vi "Design Lowpass Filter.vi"(10 "Conversion Op":T1, 11 "dt":dbl) -> (3 "filter coefficients":cluster{"beta":dbl, "gamma":dbl, "alpha":dbl} {"alpha" format="%.2f"; "gamma" format="%.2f"; "beta" format="%.2f"})   [LabVIEW 2017, in "VibrationAnalysisFunctions.lvlib"]
uses:
  <vilib>/addons/InsightCM/Utilities/Analysis/Vibration/VibrationAnalysisFunctions.lvlib
  <vilib>/addons/InsightCM/Utilities/Analysis/Shared/controls/ConversionOp.ctl
  <vilib>/addons/InsightCM/Utilities/Analysis/Shared/AnalysisHelper.lvlib
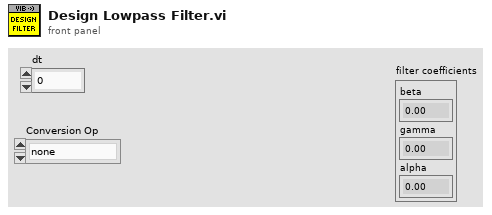
[diagram p1: front panel]
types:
  T1 = typedef "AnalysisHelper.lvlib/ConversionOp.ctl" = enum16{"none", "singleInt", "doubleInt", "singleDiff", "doubleDiff"}
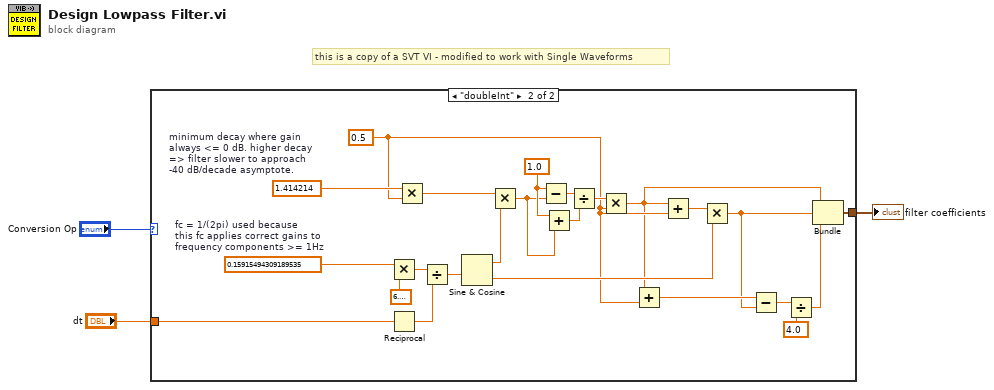
[diagram p0: block diagram]
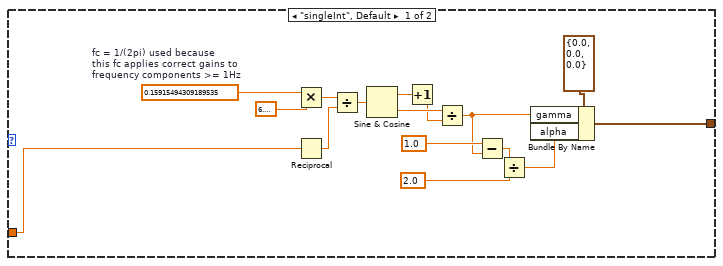
[diagram p2: hidden frame]
diagram:
  # "this is a copy of a SVT VI - modified to work with Single Waveforms"
  n1 = case shown="\"doubleInt\"" "Conversion Op" {
    tunnel: [w4 w21] -> w3
    tunnel: "dt" -> [w5 w20]
    frame "singleInt", Default {
      w19 = 0.15915494309189535  # fc = 1/(2pi) used because  this fc applies correct gains to  frequency components >= 1Hz
      n2 = Multiply(x=w19, y=6.283185307179586) -> (x*y=w13:dbl)
      n3 = Reciprocal(x=w5) -> (1/x=w14:dbl)
      n4 = Divide(x=w13, y=w14) -> (x/y=w12:dbl)
      n5 = Sine & Cosine(0:w12) -> (1:w17:dbl, 2:w16:dbl)
      n6 = Increment(x=w17) -> (x+1=w15:dbl)
      n7 = Divide(x=w16, y=w15) -> (x/y=w7:dbl)
      n8 = Subtract(x=1.0, y=w7) -> (x-y=w10:dbl)
      n9 = Divide(x=w10, y=2.0) -> (x/y=w6:dbl)
      n10 = Bundle By Name(cluster=cluster{"beta":dbl, "gamma":dbl, "alpha":dbl} {"beta"=0.0, "gamma"=0.0, "alpha"=0.0} ("filter coefficients"), "gamma"=w7, "alpha"=w6) -> (w4:cluster{"beta":dbl, "gamma":dbl, "alpha":dbl})
    }
    frame "doubleInt" {
      w25 = 0.5 ("y")
      w35 = 1.0 ("x")
      w41 = 1.414214  # minimum decay where gain  always <= 0 dB. higher decay => filter slower to approach  -40 dB/decade asymptote.
      w42 = 0.15915494309189535  # fc = 1/(2pi) used because  this fc applies correct gains to  frequency components >= 1Hz
      n11 = Multiply(x=w42, y=6.283185307179586) -> (x*y=w39:dbl)
      n12 = Reciprocal(x=w20) -> (1/x=w24:dbl)
      n13 = Multiply(x=w41, y=w25) -> (x*y=w37:dbl)
      n14 = Divide(x=w39, y=w24) -> (x/y=w38:dbl)
      n15 = Sine & Cosine(0:w38) -> (1:w36:dbl, 2:w29:dbl)
      n16 = Multiply(x=w37, y=w36) -> (x*y=w34:dbl)
      n17 = Subtract(x=w35, y=w34) -> (x-y=w33:dbl)
      n18 = Add(x=w35, y=w34) -> (x+y=w32:dbl)
      n19 = Divide(x=w33, y=w32) -> (x/y=w31:dbl)
      n20 = Multiply(x=w31, y=w25) -> (x*y=w22:dbl)
      n21 = Add(x=w22, y=w25) -> (x+y=w28:dbl)
      n22 = Add(x=w22, y=w25) -> (x+y=w30:dbl)
      n23 = Multiply(x=w30, y=w29) -> (x*y=w23:dbl)
      n24 = Subtract(x=w28, y=w23) -> (x-y=w27:dbl)
      n25 = Divide(x=w27, y=4.0) -> (x/y=w43:dbl)
      n26 = Bundle(w22, w23, w43) -> (w21:cluster{dbl, dbl, dbl})  [unwired: 1 in]
    }
  }
  "filter coefficients" <- w3
